vi "EXPORT - Invoke Command.vi"(0 "REx Command in":refnum<class "REx Command - Root.lvclass">, 7 "Session ID":string, 11 "error in (no error)":errorcluster) -> (4 "REx Command out":refnum<class "REx Command - Root.lvclass">, 15 "error out":errorcluster)   [LabVIEW 2012, in "REx.lvlib" / "Local Listener Session.lvclass"]
uses:
  Local Listener Session.lvclass
  REx Command Root/REx Command - Root.lvclass
  REx Command Root/REx Command - Root.lvclass/REx Command - Root.ctl
  Local Listener Session.lvclass/Local Listener Session.ctl
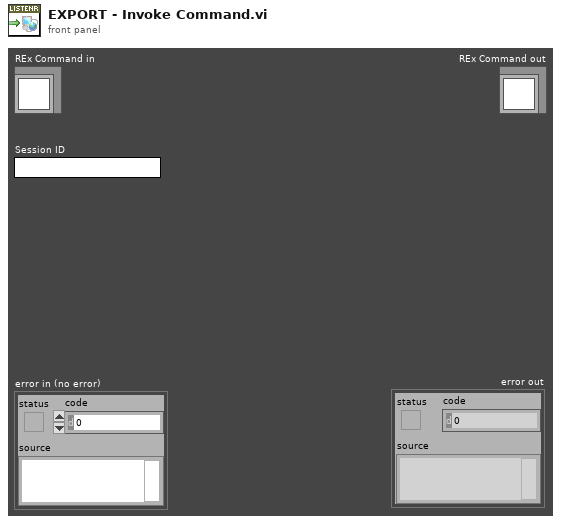
[diagram p1: front panel]
types:
  T1 = typedef "REx.lvlib/Local Listener Session.lvclass/Session Handle.ctl" = refnum<data-value>
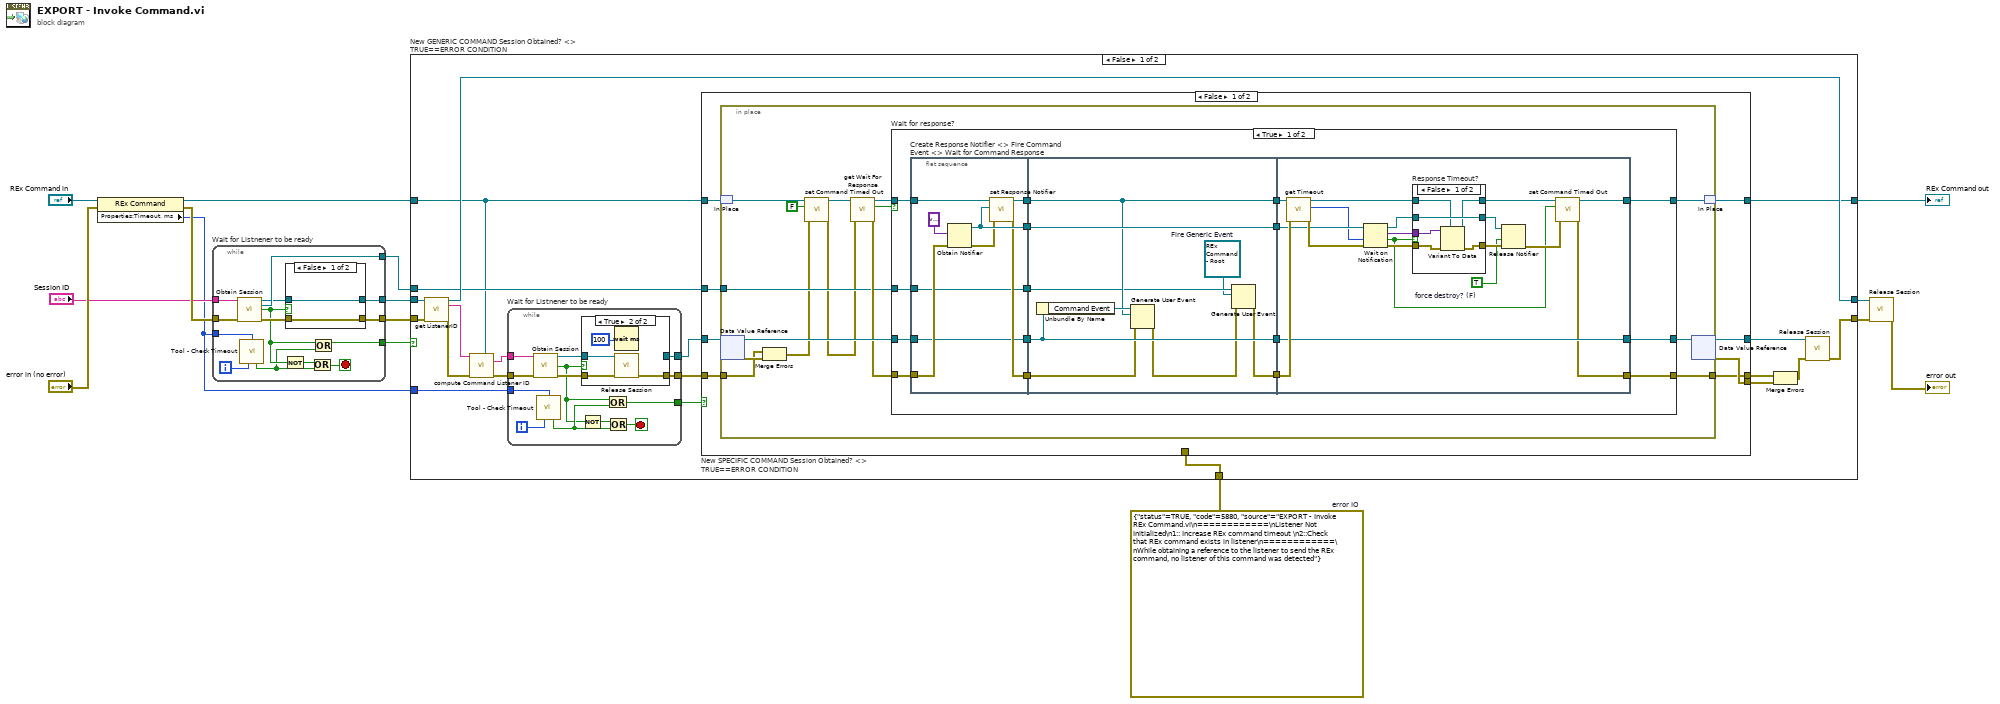
[diagram p0: block diagram]
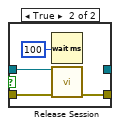
[diagram p2: hidden frame]
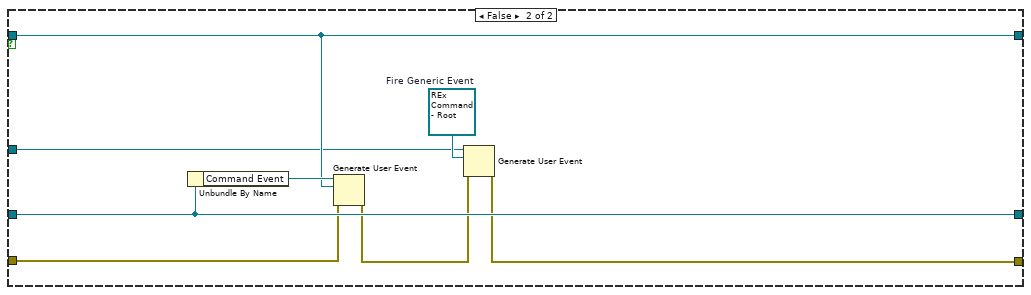
[diagram p5: hidden frame]
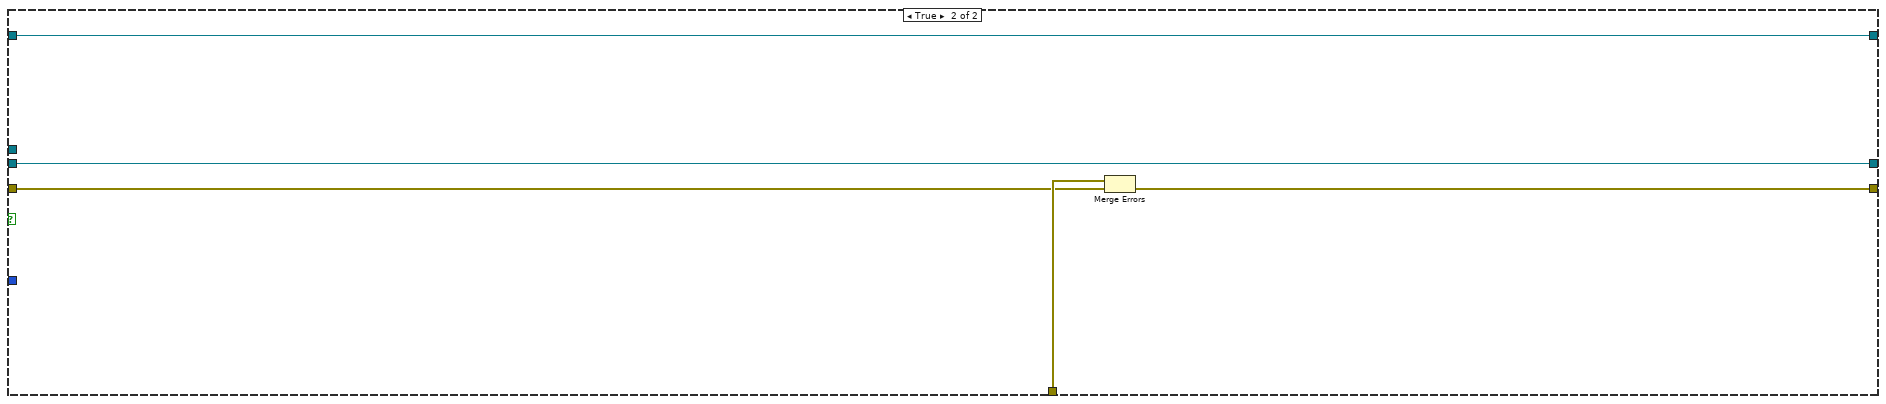
[diagram p7: hidden frame]
diagram:
  w1 = errorcluster {"status"=TRUE, "code"=5880, "source"="EXPORT - Invoke REx Command.vi\n============\nListener Not Initialized\n1:: Increase REx command timeout \n2::Check that REx command exists in listener\n============\nWhile obtaining a reference to the listener to send the REx command, no listener of this command was detected"}  # error IO
  n1 = property class="REx Command"(reference="REx Command in", error in="error in (no error)") -> (reference out=w3:refnum<class "REx Command - Root.lvclass">, error out=w14:errorcluster, "Properties:Timeout, ms"=w2:i32)
  n2 = while "Wait for Listnener to be ready" {
    tunnel: "Session ID" -> [w28]
    tunnel: [w18] -> w12
    tunnel: w14 -> [w27]
    tunnel: [w20] -> w11
    tunnel: [w26] -> w7
    tunnel: [w17] -> w5
    tunnel: w2 -> [w19]
    i -> [w23]
    stop <- w25 stop-if-true
    n3 = call "Obtain Session.vi"("Listener ID ()"=w28, "error in (no error)"=w27) -> ("Listener Session Handle"=w22:T1, "REx Command Received"=w26:refnum<user-event>, "created new?"=w17:bool, "error out"=w21:errorcluster)  [unwired: 10 in]
    n4 = call "Tool - Check Timeout.vi"("i"=w23, "Timeout, ms (10000)"=w19) -> ("Timeout?"=w16:bool)  [unwired: 12 in, 1 out]
    n5 = Not(x=w17) -> (.not. x?=w24:bool)
    n6 = case shown="False" w17 {
      tunnel: w22 -> [w30 w34]
      tunnel: w21 -> [w29 w33]
      tunnel: [w29 w32] -> w20
      tunnel: [w30 _] -> w18
      frame False {
      }
      frame True {
        n7 = Wait (ms)(milliseconds to wait=100) -> ()  [unwired: 1 out]
        n8 = call "Release Session.vi"("Session Handle"=w34, "error in (no error)"=w33) -> ("error out"=w32:errorcluster)  [unwired: 13 in]
      }
    }
    n9 = Or(x=w24, y=w16) -> (x .or. y?=w25:bool)
    n10 = Or(x=w17, y=w16) -> ()  [unwired: 1 out]
  }
  n11 = case "New GENERIC COMMAND Session Obtained? <> TRUE==ERROR CONDITION" shown="False" w5 {
    tunnel: w12 -> [w51 w173]
    tunnel: w11 -> [w50 w170]
    tunnel: [w47 w173] -> w10
    tunnel: [w46 w171] -> w9
    tunnel: w7 -> [w45 _]
    tunnel: w3 -> [w43 w174]
    tunnel: [w42 w174] -> w6
    tunnel: w2 -> [w40 _]
    tunnel: w1 -> [w35 w172]
    frame False {
      n12 = call "get ListenerID.vi"("Session Handle in"=w51, "error in (no error)"=w50) -> ("Session Handle out"=w47:T1, "Session Name"=w49:string, "error out"=w48:errorcluster)  [unwired: 11 in]
      n13 = call-dynamic "compute Command Listener ID.vi"("Listener Session ID"=w49, "REx - Command ROOT"=w43, "error in"=w48) -> ("Command Listener ID"=w38:string, "error out"=w41:errorcluster)  [unwired: 11 in]
      n14 = while "Wait for Listnener to be ready" {
        tunnel: [w60] -> w39
        tunnel: w41 -> [w67]
        tunnel: [w62] -> w37
        tunnel: [w56] -> w36
        tunnel: w40 -> [w61]
        tunnel: w38 -> [w59]
        i -> [w64]
        stop <- w66 stop-if-true
        n15 = call "Obtain Session.vi"("Listener ID ()"=w59, "error in (no error)"=w67) -> ("Listener Session Handle"=w63:T1, "created new?"=w55:bool, "error out"=w58:errorcluster)  [unwired: 10 in, 1 out]
        n16 = call "Tool - Check Timeout.vi"("i"=w64, "Timeout, ms (10000)"=w61) -> ("Timeout?"=w57:bool)  [unwired: 12 in, 1 out]
        n17 = Not(x=w55) -> (.not. x?=w65:bool)
        n18 = case shown="True" w55 {
          tunnel: w63 -> [w69 w73]
          tunnel: [w68 w72] -> w62
          tunnel: [w69 _] -> w60
          tunnel: w58 -> [w68 w71]
          frame False {
          }
          frame True {
            n19 = Wait (ms)(milliseconds to wait=100) -> ()  [unwired: 1 out]
            n20 = call "Release Session.vi"("Session Handle"=w73, "error in (no error)"=w71) -> ("error out"=w72:errorcluster)  [unwired: 13 in]
          }
        }
        n21 = Or(x=w55, y=w57) -> (x .or. y?=w56:bool)
        n22 = Or(x=w65, y=w57) -> (x .or. y?=w66:bool)
      }
      n23 = case "New SPECIFIC COMMAND Session Obtained? <> TRUE==ERROR CONDITION" shown="False" w36 {
        tunnel: w39 -> [w81 w168]
        tunnel: [w80 w168] -> w54
        tunnel: [w79 w166] -> w53
        tunnel: w45 -> [w78 _]
        tunnel: w37 -> [w77 w167]
        tunnel: [w76 w167] -> w44
        tunnel: w43 -> [w75 w169]
        tunnel: [w74 w169] -> w42
        tunnel: w35 -> [_ w166]
        frame False {
          n24 = in-place {
            in-place-border: w78 -> [w90]
            in-place-border: w77 -> [w89]
            in-place-border: [w88] -> w76
            n25 = in-place-match #1(w75) -> (w86:refnum<class "REx Command - Root.lvclass">)
            n26 = in-place-dvr #2(w81) -> (w94:refnum<class "Local Listener Session.lvclass">, w91:errorcluster)
            n27 = Merge Errors(w89, w91) -> (w85:errorcluster)
            n28 = call "set Command Timed Out.vi"("error in (no error)"=w85, "Command Timed Out?"=FALSE, "REx Command - Root in"=w86) -> ("error out"=w84:errorcluster, "REx Command - Root out"=w83:refnum<class "REx Command - Root.lvclass">)  [unwired: 7 in]
            n29 = call "get Wait For Response.vi"("error in (no error)"=w84, "REx Command - Root in"=w83) -> ("error out"=w92:errorcluster, "Wait For Response? (T)"=w95:bool, "REx Command - Root out"=w96:refnum<class "REx Command - Root.lvclass">)  [unwired: 7 in]
            n30 = case "Wait for response?" shown="True" w95 {
              tunnel: w96 -> [w112 w163]
              tunnel: [w99 w163] -> w87
              tunnel: w94 -> [w106 w164]
              tunnel: [w102 w164] -> w93
              tunnel: w92 -> [w111 w162]
              tunnel: [w100 w158] -> w88
              tunnel: w90 -> [w97 w160]
              frame True {
                n31 = flat-sequence "Create Response Notifier <> Fire Command Event <> Wait for Command Response" {
                  tunnel: w112 -> [w121]
                  tunnel: w111 -> [w118]
                  tunnel: [w120] -> w110
                  tunnel: [w119] -> w109
                  tunnel: [w117] -> w108
                  tunnel: w106 -> [w116]
                  tunnel: [w116] -> w107
                  tunnel: [w115] -> w98
                  tunnel: w97 -> [w115]
                  tunnel: w110 -> [w130]
                  tunnel: w109 -> [w127]
                  tunnel: w108 -> [w126]
                  tunnel: w107 -> [w128]
                  tunnel: [w130] -> w105
                  tunnel: [w127] -> w104
                  tunnel: [w128] -> w103
                  tunnel: [w123] -> w101
                  tunnel: w98 -> [w125]
                  tunnel: [w134] -> w99
                  tunnel: w105 -> [w146]
                  tunnel: w104 -> [w140]
                  tunnel: w103 -> [w141]
                  tunnel: [w141] -> w102
                  tunnel: w101 -> [w147]
                  tunnel: [w132] -> w100
                  frame #0 {
                    n32 = Obtain Notifier(notification data type=variant ("element data type"), error in (no error)=w118) -> (notifier out=w120:refnum<notifier>, error out=w113:errorcluster)  [unwired: 2 in, 1 out]
                    n33 = call "set Response Notifier.vi"("error in (no error)"=w113, "response notifier"=w120, "REx Command - Root in"=w121) -> ("error out"=w117:errorcluster, "REx Command - Root out"=w119:refnum<class "REx Command - Root.lvclass">)  [unwired: 7 in]
                  }
                  frame #1 {
                    w122 = refnum<class "REx Command - Root.lvclass"> refnum  # Fire Generic Event
                    n34 = Unbundle By Name(w128) -> ("Command Event"=w129:refnum<user-event>)
                    n35 = Generate User Event(user event=w129, event data cluster=w127, error in=w126) -> (error out=w124:errorcluster)  [unwired: 1 out]
                    n36 = Generate User Event(user event=w125, event data cluster=w122, error in=w124) -> (error out=w123:errorcluster)  [unwired: 1 out]
                  }
                  frame #2 {
                    w136 = TRUE  # force destroy? (F)
                    n37 = call "get Timeout.vi"("error in (no error)"=w147, "REx Command - Root in"=w140) -> ("error out"=w148:errorcluster, "timeout in ms (-1:never)"=w145:i32, "REx Command - Root out"=w144:refnum<class "REx Command - Root.lvclass">)  [unwired: 7 in]
                    n38 = Wait on Notification(notifier=w146, timeout in ms (-1)=w145, error in (no error)=w148) -> (notifier out=w139:refnum<notifier>, notification=w143:variant, timed out?=w131:bool, error out=w142:errorcluster)  [unwired: 1 in]
                    n39 = case "Response Timeout?" shown="False" w131 {
                      tunnel: w144 -> [w151 w157]
                      tunnel: w143 -> [w153 _]
                      tunnel: w142 -> [w152 w155]
                      tunnel: [w150 w157] -> w135
                      tunnel: w139 -> [w154 w156]
                      tunnel: [w154 w156] -> w138
                      tunnel: [w149 w155] -> w137
                      frame False {
                        n40 = Variant To Data(error in=w152, type=w151, Variant=w153) -> (data=w150:refnum<class "REx Command - Root.lvclass">, error out=w149:errorcluster)
                      }
                      frame True {
                      }
                    }
                    n41 = Release Notifier(notifier=w138, force destroy? (F)=w136, error in (no error)=w137) -> (error out=w133:errorcluster)  [unwired: 2 out]
                    n42 = call "set Command Timed Out.vi"("error in (no error)"=w133, "Command Timed Out?"=w131, "REx Command - Root in"=w135) -> ("error out"=w132:errorcluster, "REx Command - Root out"=w134:refnum<class "REx Command - Root.lvclass">)  [unwired: 7 in]
                  }
                }
              }
              frame False {
                w161 = refnum<class "REx Command - Root.lvclass"> refnum  # Fire Generic Event
                n43 = Unbundle By Name(w164) -> ("Command Event"=w165:refnum<user-event>)
                n44 = Generate User Event(user event=w165, event data cluster=w163, error in=w162) -> (error out=w159:errorcluster)  [unwired: 1 out]
                n45 = Generate User Event(user event=w160, event data cluster=w161, error in=w159) -> (error out=w158:errorcluster)  [unwired: 1 out]
              }
            }
            n46 = in-place-dvr #2(w93) -> (w80:T1, w79:errorcluster)
            n47 = in-place-match #1(w87) -> (w74:refnum<class "REx Command - Root.lvclass">)
          }
        }
        frame True {
        }
      }
      n48 = Merge Errors(w44, w53) -> (w52:errorcluster)
      n49 = call "Release Session.vi"("Session Handle"=w54, "error in (no error)"=w52) -> ("error out"=w46:errorcluster)  [unwired: 13 in]
    }
    frame True {
      n50 = Merge Errors(w172, w170) -> (w171:errorcluster)
    }
  }
  "REx Command out" <- w6
  n51 = call "Release Session.vi"("Session Handle"=w10, "error in (no error)"=w9) -> ("error out"=→"error out":errorcluster)  [unwired: 13 in]
